vi "ListSharedResources.vi"(7 "exact name? (F: regex)":bool, 8 "error in (no error)":errorcluster, 10 "Filter (regex|name)":string, 11 "SMO in":refnum<class "SMO.lvclass">) -> (0 "error out":errorcluster, 1 "resources found?":bool, 2 "Shared Resources":refnum<class "SMO.lvclass">[](array[class]), 3 "SMO out":refnum<class "SMO.lvclass">)   [LabVIEW 2013, in "SMO.lvclass"]
uses:
  SMO.lvclass
  <vilib>/regexp/Match Regular Expression.xnode
  Registry/Registry-SMO.lvclass
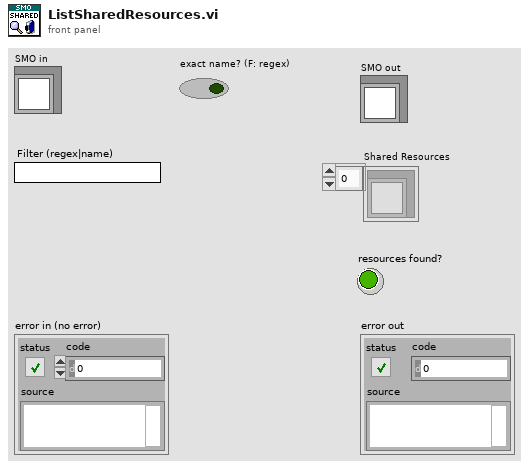
[diagram p1: front panel]
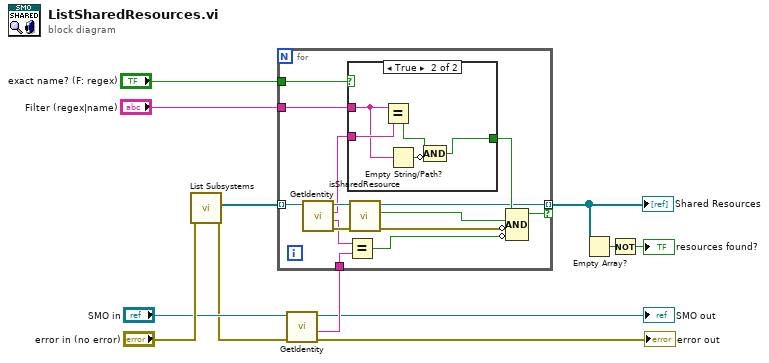
[diagram p0: block diagram]
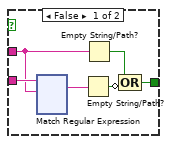
[diagram p2: hidden frame]
diagram:
  n1 = call "List Subsystems.vi"("error in (no error)"="error in (no error)") -> ("error out"=w5:errorcluster, "Subsystems"=w12:refnum<class "SMO.lvclass">[])  [unwired: 9 in]
  n2 = call "GetIdentity.vi"("error in (no error)"=w5, "SMO in"="SMO in") -> ("error out"=→"error out":errorcluster, "GUID"=w4:string, "SMO out"=→"SMO out":refnum<class "SMO.lvclass">)  [unwired: 6 in, 1 out]
  n3 = for {
    tunnel: w12 -> [w26] mode=indexing
    tunnel: [w17] -> w9 mode=indexing if=w21
    tunnel: "Filter (regex|name)" -> [w18]
    tunnel: w4 -> [w14]
    tunnel: "exact name? (F: regex)" -> [w13]
    n4 = call "GetIdentity.vi"("SMO in"=w26) -> ("error out"=w24:errorcluster, "GUID"=w15:string, "Name"=w19:string, "SMO out"=w25:refnum<class "SMO.lvclass">)  [unwired: 7 in]
    n5 = Equal?(x=w15, y=w14) -> (x = y?=w16:bool)
    n6 = case shown="True" w13 {
      tunnel: [w32 w147] -> w23
      tunnel: w19 -> [w30 w151]
      tunnel: w18 -> [w27 w149]
      frame False {
        n7 = xnode "Match Regular Expression"("input string"=w30, "regular expression"=w27) -> ("whole match"=w29:string)  [unwired: 4 in, 4 out]
        n8 = Empty String/Path?(string/path=w29) -> (empty?=w28:bool)
        n9 = Empty String/Path?(string/path=w27) -> (empty?=w31:bool)
        n10 = Compound Arithmetic op=OR(w31, invert w28) -> (w32:bool)
      }
      frame True {
        n11 = Equal?(x=w149, y=w151) -> (x = y?=w148:bool)
        n12 = Empty String/Path?(string/path=w149) -> (empty?=w150:bool)
        n13 = Compound Arithmetic op=AND(w148, invert w150) -> (w147:bool)
      }
    }
    n14 = call "isSharedResource.vi"("error in (no error)"=w24, "SMO in"=w25) -> ("error out"=w20:errorcluster, "shared resource"=w22:bool, "SMO out"=w17:refnum<class "SMO.lvclass">)  [unwired: 7 in]
    n15 = Compound Arithmetic op=AND(w23, w22, invert w20, invert w16) -> (w21:bool)
  }
  "Shared Resources" <- w9
  n16 = Empty Array?(array=w9) -> (empty?=w8:bool)
  n17 = Not(x=w8) -> (.not. x?=→"resources found?":bool)
